vi "ErrorCheckHWI.vi"(8 "error in (no error)":errorcluster, 11 "SRS_DS345 in":refnum<class "SRS_DS345.lvclass">) -> (0 "error out":errorcluster, 3 "SRS_DS345 out":refnum<class "SRS_DS345.lvclass">)   [LabVIEW 2013, in "SRS_DS345.lvclass"]
uses:
  SRS_DS345.lvclass
  SRS_DS345.lvclass/SRS_DS345.ctl
  <vilib>/Utility/error.llb/DialogType.ctl
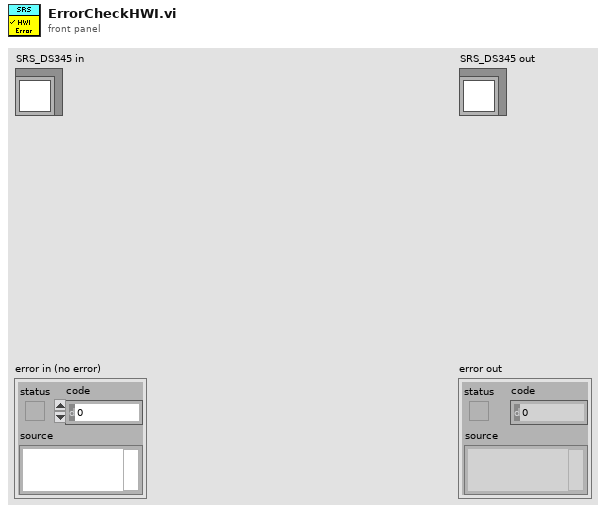
[diagram p1: front panel]
types:
  T1 = typedef "DialogType.ctl" = u16
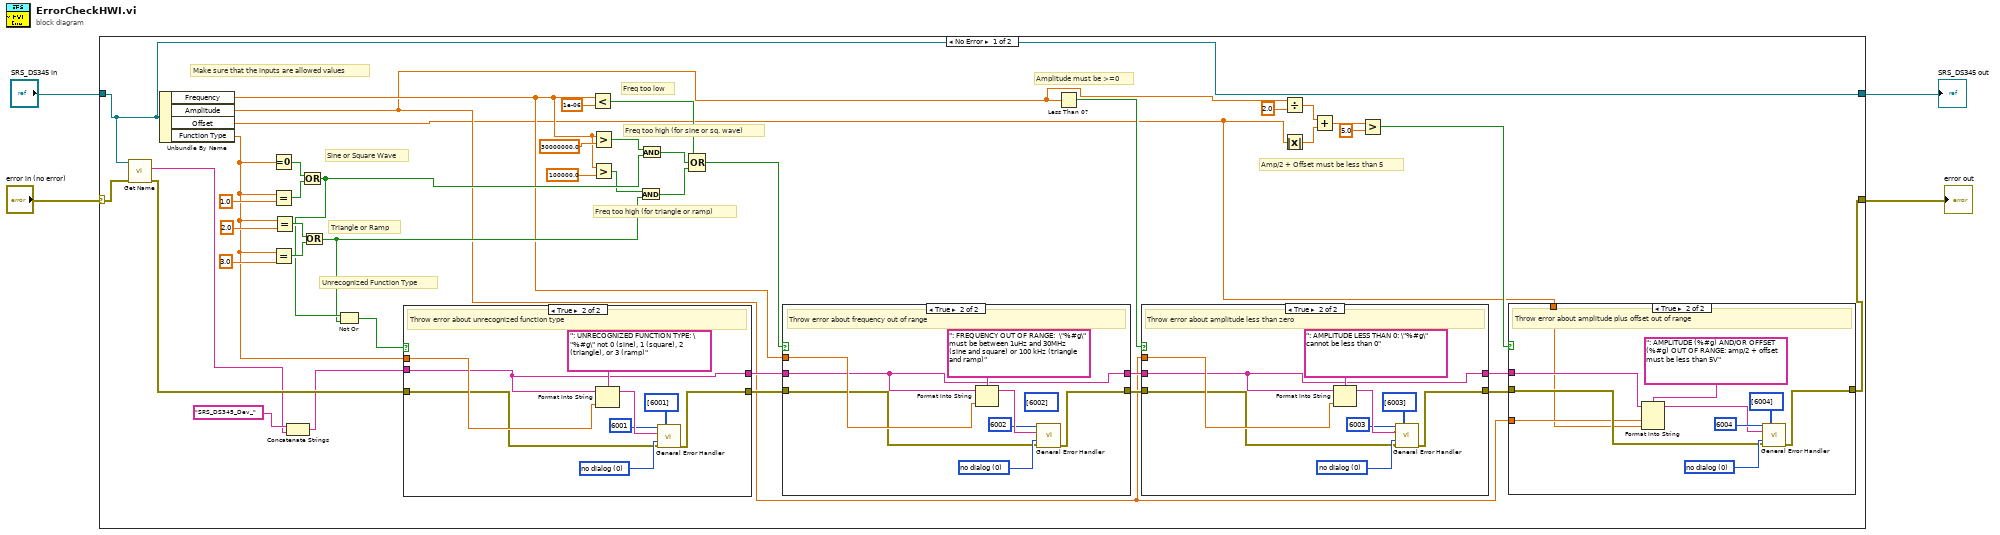
[diagram p0: block diagram]
diagram:
  n1 = case shown="No Error" "error in (no error)" {
    selector: "error in (no error)" -> [w39 w92]
    tunnel: [w8 w92] -> w1
    tunnel: "SRS_DS345 in" -> [w7 w91]
    tunnel: [w7 w91] -> w2
    frame No Error {
      # "Amp/2 + Offset must be less than 5"
      # "Amplitude must be >=0"
      # "Freq too high (for triangle or ramp)"
      # "Freq too high (for sine or sq. wave)"
      # "Freq too low"
      # "Unrecognized Function Type"
      # "Triangle or Ramp"
      # "Sine or Square Wave"
      # "Make sure that the inputs are allowed values"
      n2 = call-dynamic "Get Name.vi"("error in (no error)"=w39, "Device in"=w7) -> ("error out"=w38:errorcluster, "Name"=w23:string)  [unwired: 7 in, 1 out]
      n3 = Unbundle By Name(w7) -> ("Frequency"=w20:dbl, "Amplitude"=w6:dbl, "Offset"=w5:dbl, "Function Type"=w37:dbl)
      n4 = Equal To 0?(x=w37) -> (x = 0?=w45:bool)
      n5 = Equal?(x=w37, y=1.0) -> (x = y?=w46:bool)
      n6 = Equal?(x=w37, y=3.0) -> (x = y?=w42:bool)
      n7 = Equal?(x=w37, y=2.0) -> (x = y?=w41:bool)
      n8 = Concatenate Strings("SRS_DS345_Dev_", w23) -> (w22:string)
      n9 = Or(x=w45, y=w46) -> (x .or. y?=w32:bool)
      n10 = Or(x=w41, y=w42) -> (x .or. y?=w30:bool)
      n11 = Not Or(1:w30, 2:w32) -> (0:w40:bool)
      n12 = case shown="True" w40 {
        tunnel: w38 -> [w81 w86]
        tunnel: w22 -> [w80 w83]
        tunnel: w37 -> [_ w89]
        tunnel: [w81 w84] -> w25
        tunnel: [w80 w83] -> w21
        frame False {
        }
        frame True {
          w87 = T1 0 items=["no dialog", "OK message", "continue or stop message", "OK message + warnings", "continue/stop + warnings"] ("type of dialog (OK msg:1)")
          # "Throw error about unrecognized function type"
          n13 = Format Into String(format string=": UNRECOGNIZED FUNCTION TYPE: \"%#g\" not 0 (sine), 1 (square), 2 (triangle), or 3 (ramp)", initial string=w83, w89) -> (resulting string=w88:string)  [unwired: 1 in, 1 out]
          n14 = call <vilib>:"General Error Handler.vi"("[error code] (0)"=6001 ("error code (no error:0)"), "[user-defined codes]"=i32[] [6001], "[error source] (\" \")"=w88, "type of dialog (OK msg:1)"=w87, "error in (no error)"=w86) -> ("error out"=w84:errorcluster)  [unwired: 6 in, 4 out]
        }
      }
      n15 = Less?(x=w20, y=1e-06) -> (x < y?=w27:bool)
      n16 = Greater?(x=w20, y=30000000.0) -> (0:w33:bool)
      n17 = Greater?(x=w20, y=100000.0) -> (0:w31:bool)
      n18 = And(x=w31, y=w30) -> (x .and. y?=w29:bool)
      n19 = And(x=w33, y=w32) -> (x .and. y?=w28:bool)
      n20 = Compound Arithmetic op=OR(w27, w28, w29) -> (w26:bool)
      n21 = case shown="True" w26 {
        tunnel: w25 -> [w71 w75]
        tunnel: w20 -> [_ w78]
        tunnel: [w71 w73] -> w17
        tunnel: w21 -> [w70 w72]
        tunnel: [w70 w72] -> w18
        frame False {
        }
        frame True {
          (unwired) i32[] [6002] ("[user-defined codes]")
          w76 = T1 0 items=["no dialog", "OK message", "continue or stop message", "OK message + warnings", "continue/stop + warnings"] ("type of dialog (OK msg:1)")
          # "Throw error about frequency out of range"
          n22 = Format Into String(format string=": FREQUENCY OUT OF RANGE:  \"%#g\" must be between 1uHz and 30MHz (sine and square) or 100 kHz (triangle and ramp)", initial string=w72, w78) -> (resulting string=w77:string)  [unwired: 1 in, 1 out]
          n23 = call <vilib>:"General Error Handler.vi"("[error code] (0)"=6002 ("error code (no error:0)"), "[error source] (\" \")"=w77, "type of dialog (OK msg:1)"=w76, "error in (no error)"=w75) -> ("error out"=w73:errorcluster)  [unwired: 7 in, 4 out]
        }
      }
      n24 = Less Than 0?(x=w6) -> (x < 0?=w19:bool)
      n25 = case shown="True" w19 {
        tunnel: w17 -> [w60 w65]
        tunnel: w6 -> [_ w68]
        tunnel: [w60 w62] -> w10
        tunnel: w18 -> [w59 w61]
        tunnel: [w59 w61] -> w11
        frame False {
        }
        frame True {
          w66 = T1 0 items=["no dialog", "OK message", "continue or stop message", "OK message + warnings", "continue/stop + warnings"] ("type of dialog (OK msg:1)")
          # "Throw error about amplitude less than zero"
          n26 = Format Into String(format string=": AMPLITUDE LESS THAN 0: \"%#g\" cannot be less than 0", initial string=w61, w68) -> (resulting string=w67:string)  [unwired: 1 in, 1 out]
          n27 = call <vilib>:"General Error Handler.vi"("[error code] (0)"=6003 ("error code (no error:0)"), "[user-defined codes]"=i32[] [6003], "[error source] (\" \")"=w67, "type of dialog (OK msg:1)"=w66, "error in (no error)"=w65) -> ("error out"=w62:errorcluster)  [unwired: 6 in, 4 out]
        }
      }
      n28 = Divide(x=w6, y=2.0) -> (x/y=w15:dbl)
      n29 = Absolute Value(x=w5) -> (abs(x)=w14:dbl)
      n30 = Add(x=w15, y=w14) -> (x+y=w13:dbl)
      n31 = Greater?(x=w13, y=5.0) -> (0:w9:bool)
      n32 = case shown="True" w9 {
        tunnel: w10 -> [w48 w57]
        tunnel: [w48 w54] -> w8
        tunnel: w11 -> [_ w53]
        tunnel: w6 -> [_ w52]
        tunnel: w5 -> [_ w51]
        frame False {
        }
        frame True {
          w58 = T1 0 items=["no dialog", "OK message", "continue or stop message", "OK message + warnings", "continue/stop + warnings"] ("type of dialog (OK msg:1)")
          # "Throw error about amplitude plus offset out of range"
          n33 = Format Into String(format string=": AMPLITUDE (%#g) AND/OR OFFSET (%#g) OUT OF RANGE: amp/2 + offset must be less than 5V", initial string=w53, w52, w51) -> (resulting string=w49:string)  [unwired: 1 in, 1 out]
          n34 = call <vilib>:"General Error Handler.vi"("[error code] (0)"=6004 ("error code (no error:0)"), "[user-defined codes]"=i32[] [6004], "[error source] (\" \")"=w49, "type of dialog (OK msg:1)"=w58, "error in (no error)"=w57) -> ("error out"=w54:errorcluster)  [unwired: 6 in, 4 out]
        }
      }
    }
    frame Error {
    }
  }
  "error out" <- w1
  "SRS_DS345 out" <- w2
